vi "Find Cross.vi"(5 "Range":dbl=130.0, 7 "mm/pixel":dbl=0.4, 8 "picture":picture) -> (0 "picture":picture, 1 "mm/pixel":dbl, 2 "Range":dbl, 3 "Result":cluster{"x":dbl, "y":dbl, "a":dbl})   [LabVIEW 2013]
uses:
  <vilib>/Analysis/NI_AALPro.lvlib
panel:
  in  "path to JPEG file":path
  in  "pixel center 2":cluster{"horizontal":i16, "vertical":i16}
  in  "pixel center":cluster{"horizontal":i16, "vertical":i16}
  in  "Color":string="Red"
  in  "show?":bool=TRUE
  in  "Raw?":bool=TRUE
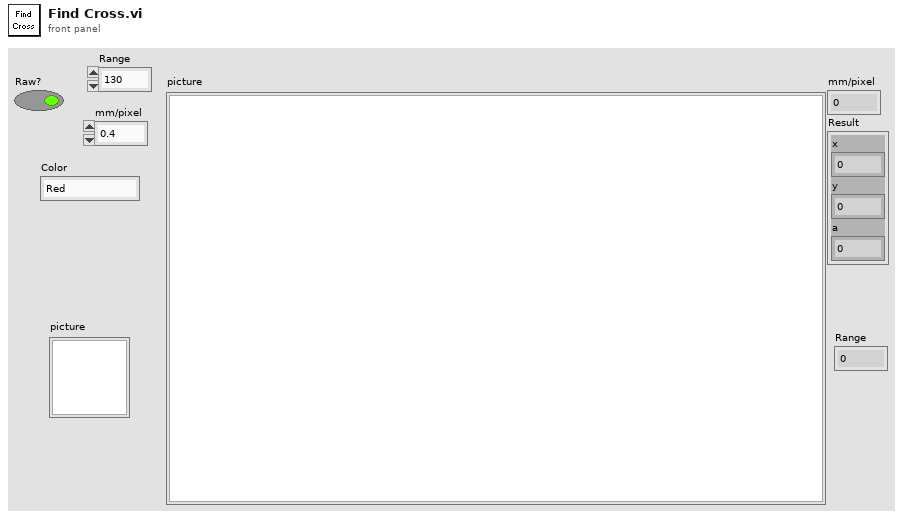
[diagram p1: front panel]
types:
  T1 = typedef "imagedata.ctl" = cluster{"image type":i32, "image depth":i32, "image":u8[], "mask":u8[], "colors":u32[], "Rectangle":cluster{"left":i16, "top":i16, "right":i16, "bottom":i16}}
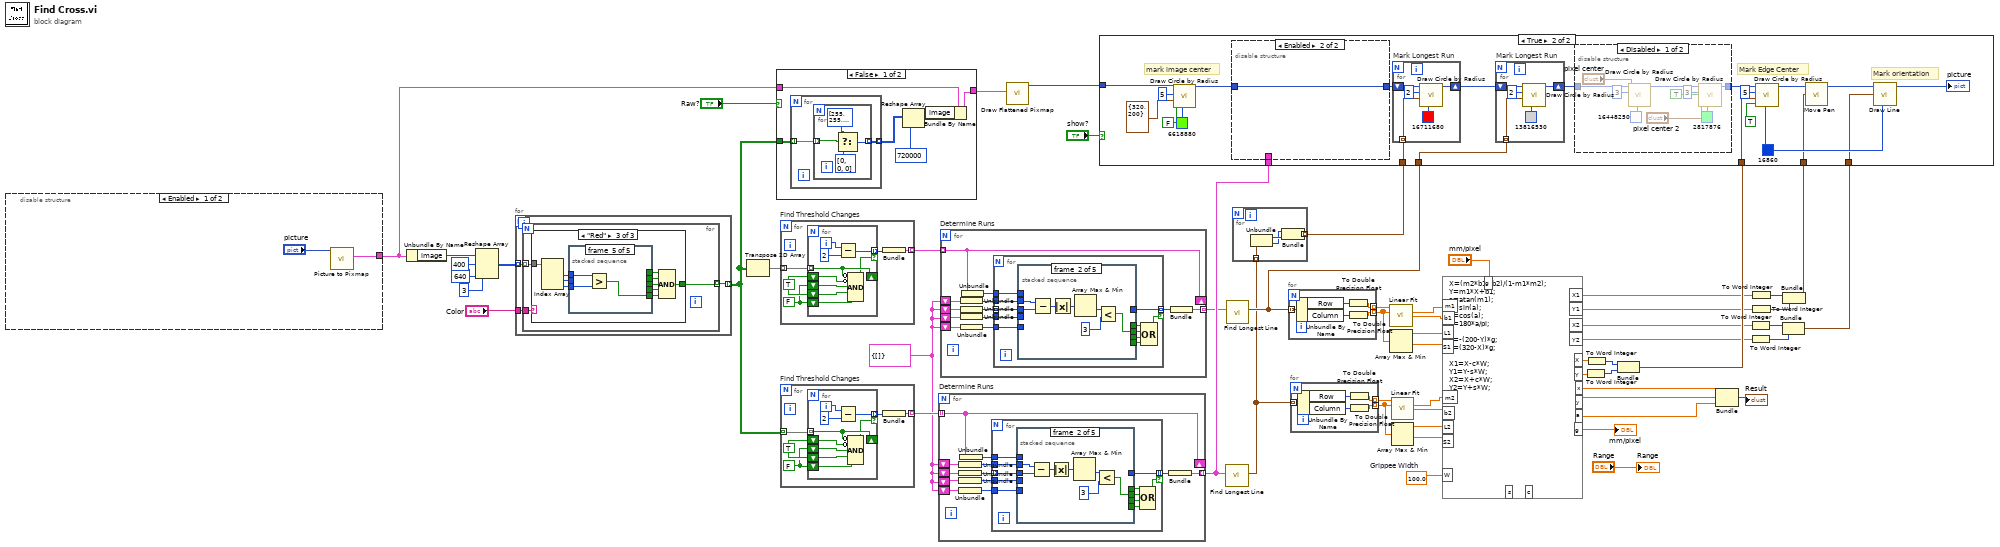
[diagram p0: block diagram]
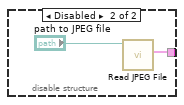
[diagram p2: hidden frame]
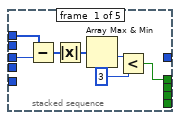
[diagram p3: hidden frame]
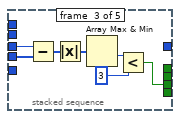
[diagram p4: hidden frame]
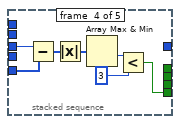
[diagram p5: hidden frame]
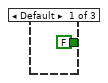
[diagram p8: hidden frame]
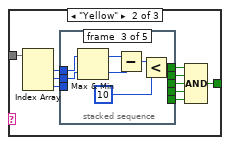
[diagram p9: hidden frame]
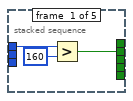
[diagram p10: hidden frame]
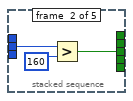
[diagram p11: hidden frame]
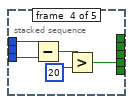
[diagram p12: hidden frame]
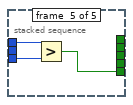
[diagram p13: hidden frame]
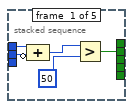
[diagram p14: hidden frame]
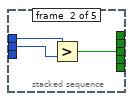
[diagram p15: hidden frame]
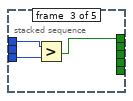
[diagram p16: hidden frame]
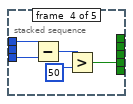
[diagram p17: hidden frame]
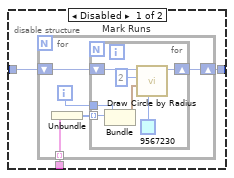
[diagram p20: hidden frame]
diagram:
  w17 = 100.0  # Grippee Width
  w35 = cluster{i32[]} {[]}
  n1 = disable-structure shown="Enabled" {
    disable-tunnel: [w58 w60] -> w51
    frame Enabled {
      n2 = call <vilib>:"Picture to Pixmap.vi"("picture"="picture") -> ("image data"=w58:T1)  [unwired: 9 in, 1 out]
    }
    frame Disabled {
      n3 = call <vilib>:"Read JPEG File.vi"("path to JPEG file"="path to JPEG file") -> ("image data"=w60:T1)  [unwired: 8 in, 2 out]
    }
  }
  n4 = Unbundle By Name(w51) -> ("image"=w52:u8[])
  n5 = Reshape Array(w52, 400 ("dimension size"), 640 ("dimension size"), 3 ("dimension size")) -> (w33:u8[][][])
  n6 = for {
    tunnel: w33 -> [w63] mode=indexing
    tunnel: [w62] -> w37 mode=indexing
    tunnel: "Color" -> [w61]
    n7 = for {
      tunnel: w63 -> [w66] mode=indexing
      tunnel: [w65] -> w62 mode=indexing
      tunnel: w61 -> [w64]
      n8 = case shown="\"Red\"" w64 {
        tunnel: w66 -> [_ w77 w108]
        tunnel: [FALSE w68 w99] -> w65
        frame Default {
        }
        frame "Yellow" {
          n9 = Index Array(array=w77) -> (element #1=w76:u8, element #2=w75:u8, element #3=w74:u8)  [unwired: 3 in]
          n10 = stacked-sequence {
            tunnel: w76 -> [w80 _ w89 w92 w97]
            tunnel: w75 -> [_ w82 w90 _ _]
            tunnel: w74 -> [_ _ _ w93 w98]
            tunnel: [_ _ _ w94 _] -> w73
            tunnel: [w78 _ _ _ _] -> w72
            tunnel: [_ w81 _ _ _] -> w71
            tunnel: [_ _ w84 _ _] -> w70
            tunnel: [_ _ _ _ w96] -> w69
            frame #0 {
              n11 = Greater?(x=w80, y=u8 160) -> (0:w78:bool)
            }
            frame #1 {
              n12 = Greater?(x=w82, y=u8 160) -> (0:w81:bool)
            }
            frame #2 {
              n13 = Max & Min(x=w89, y=w90) -> (max(x,y)=w88:u8, min(x,y)=w87:u8)
              n14 = Subtract(x=w88, y=w87) -> (x-y=w86:u8)
              n15 = Less?(x=w86, y=u8 10) -> (x < y?=w84:bool)
            }
            frame #3 {
              n16 = Subtract(x=w92, y=w93) -> (x-y=w91:u8)
              n17 = Greater?(x=w91, y=u8 20) -> (0:w94:bool)
            }
            frame #4 {
              n18 = Greater?(x=w97, y=w98) -> (0:w96:bool)
            }
          }
          n19 = Compound Arithmetic op=AND(w70, w72, w71, w73, w69) -> (w68:bool)
        }
        frame "Red" {
          n20 = Index Array(array=w108) -> (element #1=w107:u8, element #2=w106:u8, element #3=w105:u8)  [unwired: 3 in]
          n21 = stacked-sequence {
            tunnel: w107 -> [w111 w115 w118 w121 w126]
            tunnel: w106 -> [w110 w114 _ _ _]
            tunnel: w105 -> [_ _ w119 w122 w127]
            tunnel: [_ _ _ w123 _] -> w104
            tunnel: [w112 _ _ _ _] -> w103
            tunnel: [_ w116 _ _ _] -> w102
            tunnel: [_ _ w117 _ _] -> w101
            tunnel: [_ _ _ _ w125] -> w100
            frame #0 {
              n22 = Compound Arithmetic op=ADD(w111, invert w110) -> (w109:u8)
              n23 = Greater?(x=w109, y=u8 50) -> (0:w112:bool)
            }
            frame #1 {
              n24 = Greater?(x=w115, y=w114) -> (0:w116:bool)
            }
            frame #2 {
              n25 = Greater?(x=w118, y=w119) -> (0:w117:bool)
            }
            frame #3 {
              n26 = Subtract(x=w121, y=w122) -> (x-y=w120:u8)
              n27 = Greater?(x=w120, y=u8 50) -> (0:w123:bool)
            }
            frame #4 {
              n28 = Greater?(x=w126, y=w127) -> (0:w125:bool)
            }
          }
          n29 = Compound Arithmetic op=AND(w101, w103, w102, w104, w100) -> (w99:bool)
        }
      }
    }
  }
  n30 = Transpose 2D Array(2D array=w37) -> (transposed array=w50:bool[][])
  n31 = case shown="False" "Raw?" {
    tunnel: w51 -> [w133 w140]
    tunnel: [w129 w140] -> w38
    tunnel: w37 -> [w131 _]
    frame False {
      n32 = for {
        tunnel: w131 -> [w135] mode=indexing
        tunnel: [w134] -> w130 mode=indexing
        n33 = for {
          tunnel: w135 -> [w139] mode=indexing
          tunnel: [w136] -> w134 mode=indexing
          n34 = Select(t=u8[] [255, 255, 255], s=w139, f=u8[] [0, 0, 0]) -> (s? t:f=w136:u8[])
        }
      }
      n35 = Reshape Array(w130, 720000 ("dimension size")) -> (w132:u8[])
      n36 = Bundle By Name(cluster=w133, "image"=w132) -> (w129:T1)
    }
    frame True {
    }
  }
  n37 = for "Find Threshold Changes" {
    tunnel: w50 -> [w145] mode=indexing
    tunnel: [w141] -> w49 mode=indexing
    w143 = FALSE
    w144 = TRUE
    n38 = for {
      tunnel: w145 -> [w152] mode=indexing
      shift-right: [w152] -> _
      shift-left: w144 -> [w151]
      shift-left: w143 -> [w150]
      shift-left: w144 -> [w149]
      shift-left: w143 -> [w148]
      tunnel: [w147] -> w142 mode=indexing if=w146
      i -> [w154]
      n39 = Subtract(x=w154, y=2) -> (x-y=w147:i32)
      n40 = Compound Arithmetic op=AND(invert w152, invert w151, w150, w149, w148) -> (w146:bool)
    }
    n41 = Bundle(w142) -> (w141:cluster{i32[]})  [unwired: 1 in]
  }
  n42 = for "Find Threshold Changes" {
    tunnel: w37 -> [w159] mode=indexing
    tunnel: [w155] -> w36 mode=indexing
    w157 = FALSE
    w158 = TRUE
    n43 = for {
      tunnel: w159 -> [w166] mode=indexing
      shift-right: [w166] -> _
      shift-left: w158 -> [w165]
      shift-left: w157 -> [w164]
      shift-left: w158 -> [w163]
      shift-left: w157 -> [w162]
      tunnel: [w161] -> w156 mode=indexing if=w160
      i -> [w168]
      n44 = Subtract(x=w168, y=2) -> (x-y=w161:i32)
      n45 = Compound Arithmetic op=AND(invert w166, invert w165, w164, w163, w162) -> (w160:bool)
    }
    n46 = Bundle(w156) -> (w155:cluster{i32[]})  [unwired: 1 in]
  }
  n47 = for "Determine Runs" {
    tunnel: w36 -> [w179] mode=indexing
    shift-right: [w179] -> _
    shift-left: w35 -> [w178]
    shift-left: w35 -> [w180]
    shift-left: w35 -> [w177]
    shift-left: w35 -> [w176]
    tunnel: [w175] -> w32 mode=indexing
    n48 = Unbundle(w178) -> (w170:i32[])
    n49 = Unbundle(w180) -> (w171:i32[])
    n50 = Unbundle(w177) -> (w172:i32[])
    n51 = Unbundle(w176) -> (w173:i32[])
    n52 = Unbundle(w179) -> (w169:i32[])
    n53 = for {
      tunnel: w171 -> [w190] mode=indexing
      tunnel: w169 -> [w191]
      tunnel: w170 -> [w189]
      tunnel: w172 -> [w185]
      tunnel: w173 -> [w183]
      tunnel: [w182] -> w174 mode=indexing if=w181
      n54 = stacked-sequence {
        tunnel: w191 -> [w198 _ _ _ _]
        tunnel: w190 -> [w197 w205 w207 w215 w220]
        tunnel: w189 -> [_ w200 _ _ _]
        tunnel: [_ w199 _ _ _] -> w188
        tunnel: [w192 _ _ _ _] -> w187
        tunnel: [_ _ w208 _ _] -> w186
        tunnel: w185 -> [_ _ w206 _ _]
        tunnel: [_ _ _ w214 _] -> w184
        tunnel: w183 -> [_ _ _ w213 _]
        tunnel: [_ _ _ _ w220] -> w182
        frame #0 {
          n55 = Subtract(x=w198, y=w197) -> (x-y=w196:i32[])
          n56 = Absolute Value(x=w196) -> (abs(x)=w195:i32[])
          n57 = Array Max & Min(array=w195) -> (min value=w194:i32)  [unwired: 3 out]
          n58 = Less?(x=w194, y=3) -> (x < y?=w192:bool)
        }
        frame #1 {
          n59 = Subtract(x=w200, y=w205) -> (x-y=w204:i32[])
          n60 = Absolute Value(x=w204) -> (abs(x)=w203:i32[])
          n61 = Array Max & Min(array=w203) -> (min value=w202:i32)  [unwired: 3 out]
          n62 = Less?(x=w202, y=3) -> (x < y?=w199:bool)
        }
        frame #2 {
          n63 = Subtract(x=w207, y=w206) -> (x-y=w212:i32[])
          n64 = Absolute Value(x=w212) -> (abs(x)=w211:i32[])
          n65 = Array Max & Min(array=w211) -> (min value=w210:i32)  [unwired: 3 out]
          n66 = Less?(x=w210, y=3) -> (x < y?=w208:bool)
        }
        frame #3 {
          n67 = Subtract(x=w215, y=w213) -> (x-y=w219:i32[])
          n68 = Absolute Value(x=w219) -> (abs(x)=w218:i32[])
          n69 = Array Max & Min(array=w218) -> (min value=w217:i32)  [unwired: 3 out]
          n70 = Less?(x=w217, y=3) -> (x < y?=w214:bool)
        }
        frame #4 {
        }
      }
      n71 = Compound Arithmetic op=OR(w187, w188, w186, w184) -> (w181:bool)
    }
    n72 = Bundle(w174) -> (w175:cluster{i32[]})  [unwired: 1 in]
  }
  n73 = for "Determine Runs" {
    tunnel: w49 -> [w231] mode=indexing
    shift-right: [w231] -> _
    shift-left: w35 -> [w230]
    shift-left: w35 -> [w232]
    shift-left: w35 -> [w229]
    shift-left: w35 -> [w228]
    tunnel: [w227] -> w31 mode=indexing
    n74 = Unbundle(w230) -> (w222:i32[])
    n75 = Unbundle(w232) -> (w223:i32[])
    n76 = Unbundle(w229) -> (w224:i32[])
    n77 = Unbundle(w228) -> (w225:i32[])
    n78 = Unbundle(w231) -> (w221:i32[])
    n79 = for {
      tunnel: w223 -> [w242] mode=indexing
      tunnel: w221 -> [w243]
      tunnel: w222 -> [w241]
      tunnel: w224 -> [w237]
      tunnel: w225 -> [w235]
      tunnel: [w234] -> w226 mode=indexing if=w233
      n80 = stacked-sequence {
        tunnel: w243 -> [w250 _ _ _ _]
        tunnel: w242 -> [w249 w257 w259 w267 w272]
        tunnel: w241 -> [_ w252 _ _ _]
        tunnel: [_ w251 _ _ _] -> w240
        tunnel: [w244 _ _ _ _] -> w239
        tunnel: [_ _ w260 _ _] -> w238
        tunnel: w237 -> [_ _ w258 _ _]
        tunnel: [_ _ _ w266 _] -> w236
        tunnel: w235 -> [_ _ _ w265 _]
        tunnel: [_ _ _ _ w272] -> w234
        frame #0 {
          n81 = Subtract(x=w250, y=w249) -> (x-y=w248:i32[])
          n82 = Absolute Value(x=w248) -> (abs(x)=w247:i32[])
          n83 = Array Max & Min(array=w247) -> (min value=w246:i32)  [unwired: 3 out]
          n84 = Less?(x=w246, y=3) -> (x < y?=w244:bool)
        }
        frame #1 {
          n85 = Subtract(x=w252, y=w257) -> (x-y=w256:i32[])
          n86 = Absolute Value(x=w256) -> (abs(x)=w255:i32[])
          n87 = Array Max & Min(array=w255) -> (min value=w254:i32)  [unwired: 3 out]
          n88 = Less?(x=w254, y=3) -> (x < y?=w251:bool)
        }
        frame #2 {
          n89 = Subtract(x=w259, y=w258) -> (x-y=w264:i32[])
          n90 = Absolute Value(x=w264) -> (abs(x)=w263:i32[])
          n91 = Array Max & Min(array=w263) -> (min value=w262:i32)  [unwired: 3 out]
          n92 = Less?(x=w262, y=3) -> (x < y?=w260:bool)
        }
        frame #3 {
          n93 = Subtract(x=w267, y=w265) -> (x-y=w271:i32[])
          n94 = Absolute Value(x=w271) -> (abs(x)=w270:i32[])
          n95 = Array Max & Min(array=w270) -> (min value=w269:i32)  [unwired: 3 out]
          n96 = Less?(x=w269, y=3) -> (x < y?=w266:bool)
        }
        frame #4 {
        }
      }
      n97 = Compound Arithmetic op=OR(w239, w240, w238, w236) -> (w233:bool)
    }
    n98 = Bundle(w226) -> (w227:cluster{i32[]})  [unwired: 1 in]
  }
  n99 = call <vilib>:"Draw Flattened Pixmap.vi"("image data"=w38) -> ("new picture"=w53:picture)  [unwired: 8 in]
  n100 = call "Find Longest Line.vi"("Array"=w32) -> ("Edge"=w27:cluster{"Column":i32, "Row":i32}[])  [unwired: 10 in]
  n101 = call "Find Longest Line.vi"("Array"=w31) -> ("Edge"=w30:cluster{"Column":i32, "Row":i32}[])  [unwired: 10 in]
  n102 = for {
    tunnel: w27 -> [w276] mode=indexing
    tunnel: [w273] -> w34 mode=indexing
    n103 = Unbundle(w276) -> ("Column"=w275:i32, "Row"=w274:i32)
    n104 = Bundle("Row"=w274, "Column"=w275) -> (w273:cluster{"Row":i32, "Column":i32})  [unwired: 1 in]
  }
  n105 = for {
    tunnel: w30 -> [w279] mode=indexing
    tunnel: [w278] -> w42 mode=indexing
    tunnel: [w277] -> w40 mode=indexing
    n106 = Unbundle By Name(w279) -> ("Row"=w280:i32, "Column"=w281:i32)
    n107 = To Double Precision Float(number=w280) -> (double precision float=w278:dbl)
    n108 = To Double Precision Float(number=w281) -> (double precision float=w277:dbl)
  }
  n109 = for {
    tunnel: [w282] -> _ mode=indexing
    tunnel: [w284] -> w29 mode=indexing
    tunnel: [w283] -> w28 mode=indexing
    tunnel: w27 -> [w282] mode=indexing
    n110 = Unbundle By Name(w282) -> ("Row"=w285:i32, "Column"=w286:i32)
    n111 = To Double Precision Float(number=w285) -> (double precision float=w284:dbl)
    n112 = To Double Precision Float(number=w286) -> (double precision float=w283:dbl)
  }
  n113 = call <vilib>:"Linear Fit.vi"("Y"=w42, "X"=w40) -> ("slope"=w25:dbl, "intercept"=w26:dbl)  [unwired: 9 in, 3 out]
  n114 = Array Max & Min(array=w40) -> (max value=w20:dbl, min value=w19:dbl)  [unwired: 2 out]
  n115 = call <vilib>:"Linear Fit.vi"("Y"=w29, "X"=w28) -> ("slope"=w23:dbl, "intercept"=w24:dbl)  [unwired: 9 in, 3 out]
  n116 = Array Max & Min(array=w28) -> (max value=w22:dbl, min value=w21:dbl)  [unwired: 2 out]
  n117 = formula code="X=(m2*b1+b2)/(1-m1*m2);\nY=m1*X+b1;\na=atan(m1);\ns=sin(a);\nc=cos(a);\na=180*a/pi;\n\nx=-(200-Y)*g;\ny=(320-X)*g;\n\nX1=X-c*W;\nY1=Y-s*W;\nX2=X+c*W;\nY2=Y+s*W;"("m1"=w25, "b1"=w26, "b2"=w24, "m2"=w23, "L2"=w22, "S2"=w21, "L1"=w20, "S1"=w19, "W"=w17, "g"="mm/pixel") -> ("x"=w15:dbl, "y"=w16:dbl, "a"=w14:dbl, "g"=→"mm/pixel":dbl, "X"=w13:dbl, "Y"=w12:dbl, "X1"=w11:dbl, "Y1"=w10:dbl, "X2"=w7:dbl, "Y2"=w6:dbl)  [unwired: 2 out]
  n118 = To Word Integer(number=w12) -> (16bit integer=w44:i16)
  n119 = To Word Integer(number=w13) -> (16bit integer=w45:i16)
  n120 = Bundle(w45, w44) -> (w43:cluster{i16, i16})  [unwired: 1 in]
  n121 = Bundle("x"=w15, "y"=w16, "a"=w14) -> (→"Result":cluster{"x":dbl, "y":dbl, "a":dbl})  [unwired: 1 in]
  n122 = To Word Integer(number=w7) -> (16bit integer=w9:i16)
  n123 = To Word Integer(number=w6) -> (16bit integer=w8:i16)
  n124 = To Word Integer(number=w11) -> (16bit integer=w48:i16)
  n125 = To Word Integer(number=w10) -> (16bit integer=w47:i16)
  n126 = Bundle(w9, w8) -> (w5:cluster{i16, i16})  [unwired: 1 in]
  n127 = Bundle(w48, w47) -> (w46:cluster{i16, i16})  [unwired: 1 in]
  n128 = case shown="True" "show?" {
    tunnel: w53 -> [_ w308]
    tunnel: w32 -> [_ w303]
    tunnel: w46 -> [_ w290]
    tunnel: w43 -> [_ w296]
    tunnel: w34 -> [_ w295]
    tunnel: w30 -> [_ w292]
    tunnel: w5 -> [_ w289]
    frame False {
    }
    frame True {
      w294 = u32 16860
      # "Mark orientation"
      # "Mark Edge Center"
      # "mark image center"
      n129 = call <vilib>:"Draw Circle by Radius.vi"("color(black)"=u32 6618880, "fill?(F)"=FALSE, "pixel center"=cluster{"horizontal":i16, "vertical":i16} {"horizontal"=320, "vertical"=200}, "radius"=i16 5, "picture"=w308) -> ("new picture"=w302:picture)  [unwired: 6 in]
      n130 = disable-structure shown="Enabled" {
        disable-tunnel: w303 -> [w322 _]
        disable-tunnel: w302 -> [w321 w335]
        disable-tunnel: [w320 w335] -> w301
        frame Disabled {
          n131 = for "Mark Runs" {
            shift-right: [w326] -> w320
            shift-left: w321 -> [w327]
            tunnel: w322 -> [w325] mode=indexing
            i -> [w323]
            n132 = Unbundle(w325) -> (w324:i32[])
            n133 = for {
              tunnel: w324 -> [w331] mode=indexing
              shift-right: [w333] -> w326
              shift-left: w327 -> [w334]
              tunnel: w323 -> [w328]
              n134 = Bundle(w331, w328) -> (w330:cluster{i32, i32})  [unwired: 1 in]
              n135 = call <vilib>:"Draw Circle by Radius.vi"("color(black)"=u32 9567230, "pixel center"=w330, "radius"=i16 2, "picture"=w334) -> ("new picture"=w333:picture)  [unwired: 7 in]
            }
          }
        }
        frame Enabled {
        }
      }
      n136 = for "Mark Longest Run" {
        shift-right: [w344] -> w293
        shift-left: w301 -> [w345]
        tunnel: w295 -> [w341] mode=indexing
        n137 = call <vilib>:"Draw Circle by Radius.vi"("color(black)"=u32 16711680, "pixel center"=w341, "radius"=i16 2, "picture"=w345) -> ("new picture"=w344:picture)  [unwired: 7 in]
      }
      n138 = for "Mark Longest Run" {
        shift-right: [w339] -> w288
        shift-left: w293 -> [w340]
        tunnel: w292 -> [w336] mode=indexing
        n139 = call <vilib>:"Draw Circle by Radius.vi"("color(black)"=u32 13816530, "pixel center"=w336, "radius"=i16 2, "picture"=w340) -> ("new picture"=w339:picture)  [unwired: 7 in]
      }
      n140 = disable-structure shown="Disabled" {
        disable-tunnel: w288 -> [w317 w319]
        disable-tunnel: [w311 w319] -> w287
        frame Disabled {
          n141 = call <vilib>:"Draw Circle by Radius.vi"("color(black)"=u32 16448250, "pixel center"="pixel center", "radius"=i16 3, "picture"=w317) -> ("new picture"=w312:picture)  [unwired: 7 in]
          n142 = call <vilib>:"Draw Circle by Radius.vi"("color(black)"=u32 2817876, "fill?(F)"=TRUE, "pixel center"="pixel center 2", "radius"=i16 3, "picture"=w312) -> ("new picture"=w311:picture)  [unwired: 6 in]
        }
        frame Enabled {
        }
      }
      n143 = call <vilib>:"Draw Circle by Radius.vi"("color(black)"=w294, "fill?(F)"=TRUE, "pixel center"=w296, "radius"=i16 5, "picture"=w287) -> ("new picture"=w298:picture)  [unwired: 6 in]
      n144 = call <vilib>:"Move Pen.vi"("new position"=w290, "picture"=w298) -> ("new picture"=w297:picture)  [unwired: 3 in]
      n145 = call <vilib>:"Draw Line.vi"("picture"=w297, "end point"=w289, "color(black)"=w294) -> ("new picture"=→"picture":picture)  [unwired: 6 in]
    }
  }
  "Range" <- "Range"
